vi "DB Panel init.vi"(7 "Stations":cluster{"Stations":string, "alias":string}[](array[cluster]), 8 "error in (no error)":errorcluster, 9 "Line_Name":string, 10 "Table":cluster{"Table":string, "alias":string}[](array[cluster]), 11 "Ctr.DB Dispaly":refnum<vi>) -> (0 "error out":errorcluster)   [LabVIEW 2014]
uses:
  Type'def/DB Query.ctl
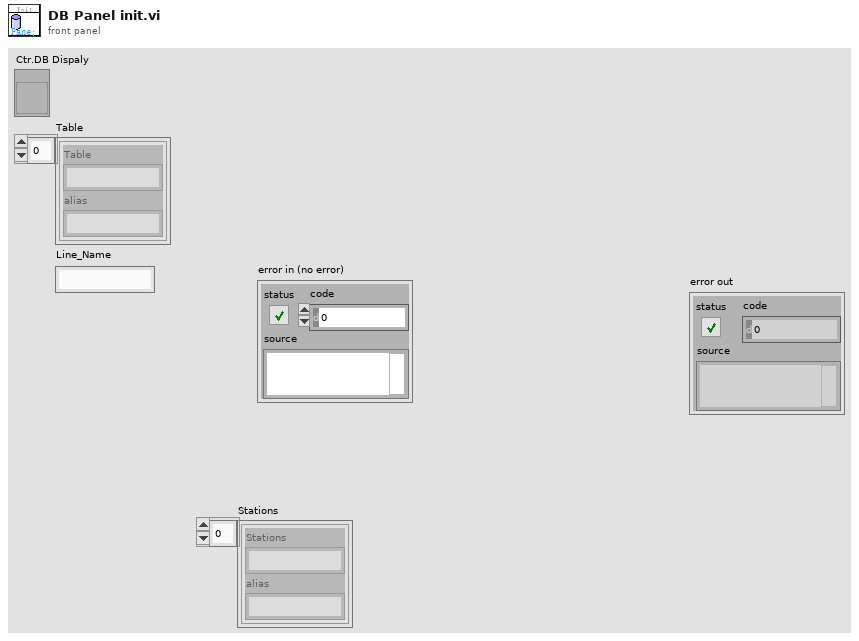
[diagram p1: front panel]
types:
  T1 = typedef "DB Query.ctl" = cluster{"Export":bool, "Query":bool, "Station.No":string, "EndTime":timestamp, "StartTime":timestamp, "FTT":cluster{"FTT":string, "OutLine":string, "FTT Rata":string}, "TableName":string, "List":string[][], "Station":bool, "QTime":enum32{"Online", "Outline"}}
  T2 = typedef "LVDateTimeRec.ctl" = cluster{"fractional second":dbl, "second":i32, "minute":i32, "hour":i32, "day of month":i32, "month":i32, "year":i32, "day of week":i32, "day of year":i32, "DST":i32}
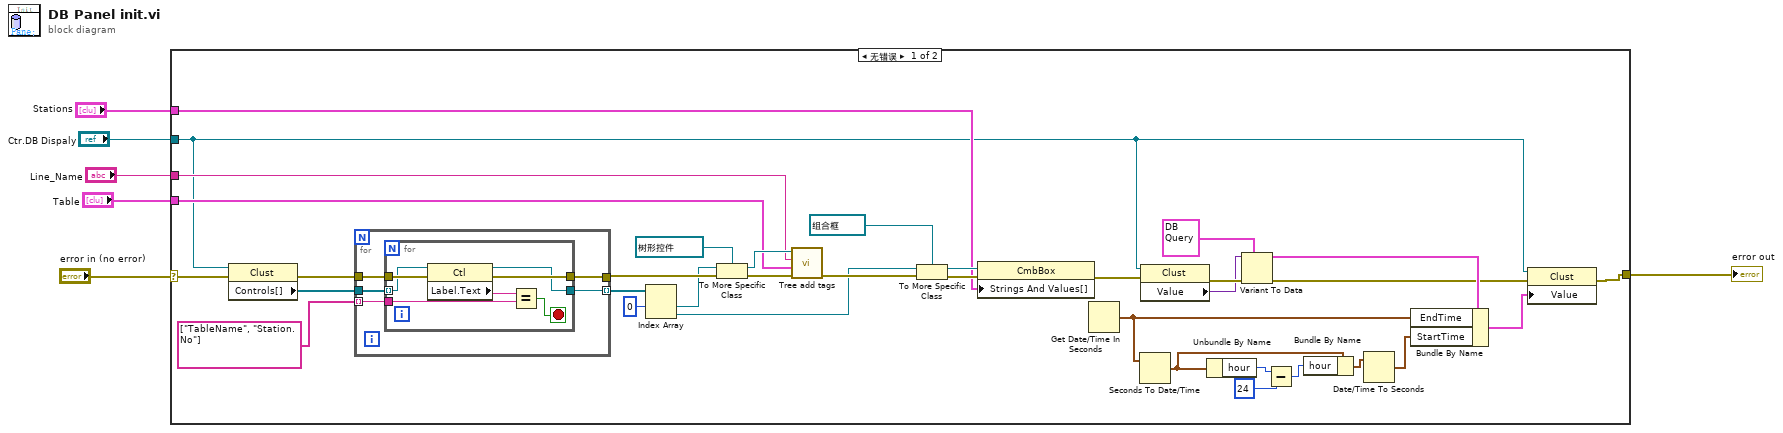
[diagram p0: block diagram]
diagram:
  n1 = case shown="无错误" "error in (no error)" {
    selector: "error in (no error)" -> [w41 w54]
    tunnel: "Ctr.DB Dispaly" -> [w9 _]
    tunnel: "Table" -> [w30 _]
    tunnel: "Line_Name" -> [w29 _]
    tunnel: "Stations" -> [w23 _]
    tunnel: [w8 w54] -> w1
    frame No Error {
      n2 = property class="Clust"(reference=w9, error in=w41) -> (error out=w39:errorcluster, "Controls[]"=w40:refnum<vi>[])  [unwired: 1 out]
      n3 = for {
        tunnel: w40 -> [w45]
        tunnel: w39 -> [w46]
        tunnel: string[] ["TableName", "Station.No"] -> [w44] mode=indexing
        tunnel: [w43] -> w37 mode=indexing
        tunnel: [w42] -> w35
        n4 = for {
          tunnel: w46 -> [w53]
          tunnel: w45 -> [w52] mode=indexing
          tunnel: w44 -> [w51]
          tunnel: [w47] -> w43
          tunnel: [w48] -> w42
          stop <- w50 stop-if-true
          n5 = property class="Ctl"(reference=w52, error in=w53) -> (reference out=w47:refnum<vi>, error out=w48:errorcluster, "Label.Text"=w49:string)
          n6 = Equal?(x=w49, y=w51) -> (x = y?=w50:bool)
        }
      }
      n7 = Index Array(array=w37, index #1=0 ("index")) -> (element #1=w34:refnum<vi>, element #2=w27:refnum<vi>)  [unwired: 1 in]
      n8 = To More Specific Class(target class=refnum<vi> refnum ("element"), reference=w34, error in=w35) -> (specific class reference=w31:refnum<vi>, error out=w32:errorcluster)
      n9 = call "Tree add tags.vi"("error in (no error)"=w32, "Table"=w30, "Line_Name"=w29, "specific class reference"=w31) -> ("error out"=w28:errorcluster)  [unwired: 6 in, 1 out]
      n10 = To More Specific Class(target class=refnum<vi> refnum ("element"), reference=w27, error in=w28) -> (specific class reference=w24:refnum<vi>, error out=w26:errorcluster)
      n11 = property class="CmbBox"(reference=w24, error in=w26, "Strings And Values[]"=w23) -> (error out=w22:errorcluster)  [unwired: 1 out]
      n12 = Get Date/Time In Seconds() -> (seconds since 1Jan1904=w17:timestamp)
      n13 = Seconds To Date/Time(time stamp (now)=w17) -> (date time rec=w16:T2)  [unwired: 1 in]
      n14 = property class="Clust"(reference=w9, error in=w22) -> (error out=w21:errorcluster, "Value"=w20:variant)  [unwired: 1 out]
      n15 = Unbundle By Name(w16) -> ("hour"=w15:i32)
      n16 = Variant To Data(error in=w21, type=T1 {"Export"=FALSE, "Query"=FALSE, "Station.No"="", "EndTime"=timestamp(0 s since 1904-01-01), "StartTime"=timestamp(0 s since 1904-01-01), "FTT"={"FTT"="", "OutLine"="", "FTT Rata"=""}, "TableName"="", "List"=[], "Station"=FALSE, "QTime"=enum."Online"} ("DB Dispaly"), Variant=w20) -> (data=w18:T1, error out=w10:errorcluster)
      n17 = Subtract(x=w15, y=24) -> (x-y=w13:i32)
      n18 = Bundle By Name(cluster=w16, "hour"=w13) -> (w12:T2)
      n19 = Date/Time To Seconds(2:w12) -> (0:w11:timestamp)  [unwired: 1 in]
      n20 = Bundle By Name(cluster=w18, "EndTime"=w17, "StartTime"=w11) -> (w7:T1)
      n21 = property class="Clust"(reference=w9, error in=w10, "Value"=w7) -> (error out=w8:errorcluster)  [unwired: 1 out]
    }
    frame Error {
    }
  }
  "error out" <- w1
